vi "Step Get All.vi"(8 "error in (no error)":errorcluster, 9 "All Steps? (f)":bool, 10 "sxSequenceId":string, 11 "Connection Refnum":T1) -> (0 "error out":errorcluster, 1 "Any Quickmode Allowed?":bool, 2 "Sequence Steps":T2[](array[typedef]), 3 "Connection Refnum":T1, 4 "Data Present":bool)   [LabVIEW 2011]
uses:
  Step Record.ctl
  Summitek EXT/ODBC/SQL Controls/Connection Refnum.ctl
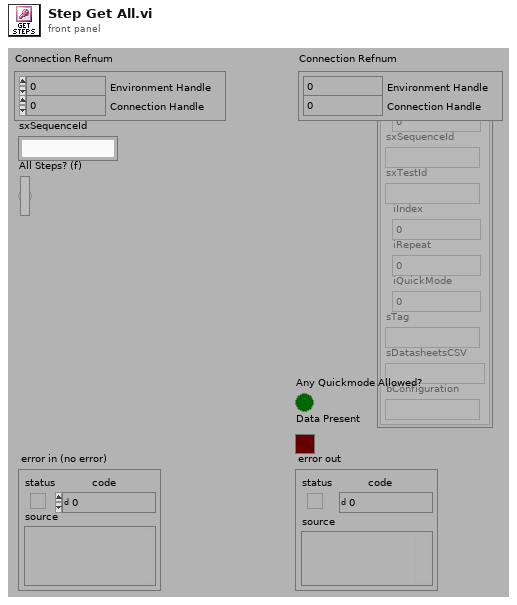
[diagram p1: front panel]
types:
  T1 = typedef "Connection Refnum.ctl" = cluster{"Environment Handle":i32, "Connection Handle":i32}
  T2 = typedef "Step Record.ctl" = cluster{"ixStep":i32, "sxSequenceId":string, "sxTestId":string, "iIndex":i32, "iRepeat":i32, "iQuickMode":i32, "sTag":string, "sDatasheetsCSV":string, "bConfiguration":string}
  T3 = typedef "Statement Refnum.ctl" = cluster{"Statement Handle":i32, "Parameter Number":u16}
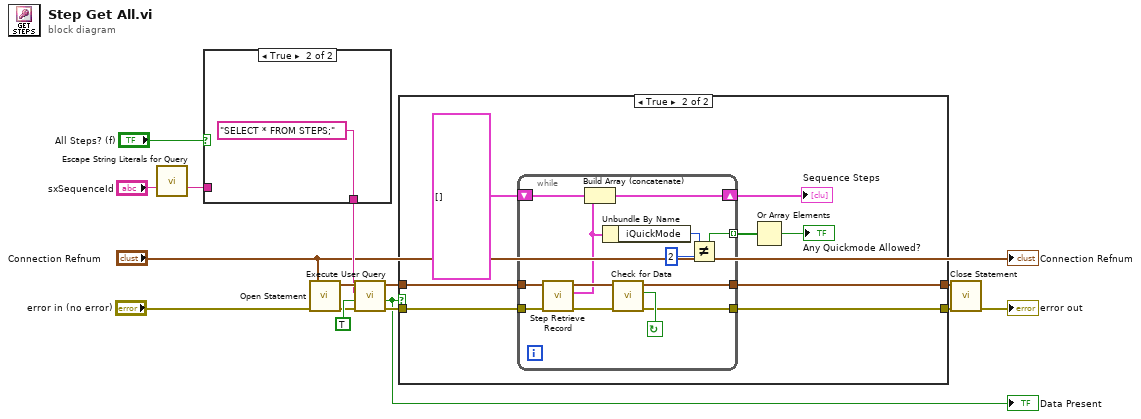
[diagram p0: block diagram]
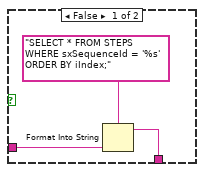
[diagram p2: hidden frame]
diagram:
  n1 = call "Escape String Literals for Query.vi"("String"="sxSequenceId") -> ("escaped String"=w4:string)  [unwired: 1 in, 13 out]
  n2 = case shown="True" "All Steps? (f)" {
    tunnel: w4 -> [w17 _]
    tunnel: [w16 "SELECT * FROM STEPS;" ("User Query")] -> w8
    frame False {
      n3 = Format Into String(format string="SELECT * FROM STEPS WHERE sxSequenceId = '%s' ORDER BY iIndex;" ("User Query"), w17) -> (resulting string=w16:string)  [unwired: 2 in, 1 out]
    }
    frame True {
    }
  }
  n4 = call "Open Statement.vi"("error in (no error)"="error in (no error)", "Connection Refnum"="Connection Refnum") -> ("error out"=w9:errorcluster, "Statement Refnum"=w10:T3)  [unwired: 4 out]
  n5 = call "Execute User Query.vi"("error in (no error)"=w9, "Return Data? (f)"=TRUE, "User Query"=w8, "Statement Refnum"=w10) -> ("error out"=w15:errorcluster, "Data Present?"=w7:bool, "Statement Refnum"=w14:T3)  [unwired: 1 out]
  "Data Present" <- w7
  n6 = case shown="True" w7 {
    tunnel: w15 -> [w20 w28]
    tunnel: w14 -> [w21 w29]
    tunnel: [w20 w26] -> w11
    tunnel: [w21 w27] -> w12
    frame False {
    }
    frame True {
      n7 = while {
        tunnel: w29 -> [w39]
        tunnel: w28 -> [w38]
        tunnel: [w36] -> w27
        tunnel: [w34] -> w26
        shift-right: [w42] -> w24
        shift-left: T2[] [] -> [w41]
        tunnel: [w30] -> w23 mode=indexing
        stop <- w40 continue-if-true
        n8 = call "Step Retrieve Record.vi"("error in (no error)"=w38, "Statement Refnum"=w39) -> ("error out"=w35:errorcluster, "Step"=w33:T2, "Statement Refnum"=w37:T3)  [unwired: 7 out]
        n9 = Build Array (concatenate)(w41, w33) -> (w42:T2[])
        n10 = Unbundle By Name(w33) -> ("iQuickMode"=w32:i32)
        n11 = call "Check for Data.vi"("error in (no error)"=w35, "Statement Refnum"=w37) -> ("error out"=w34:errorcluster, "Data Present?"=w40:bool, "Statement Refnum"=w36:T3)  [unwired: 3 out]
        n12 = Not Equal?(x=w32, y=2) -> (x != y?=w30:bool)
      }
      "Sequence Steps" <- w24
      n13 = Or Array Elements(Boolean array=w23) -> (logical OR=→"Any Quickmode Allowed?":bool)
    }
  }
  n14 = call "Close Statement.vi"("error in (no error)"=w11, "Statement Refnum"=w12) -> ("error out"=→"error out":errorcluster)  [unwired: 5 out]
  "Connection Refnum" <- "Connection Refnum"
